vi "Get 3-Rayleigh Parameters(SubVI).vi"(6 "Flow Peak Amp.":dbl, 8 "T_Flow Start (s)":dbl, 9 "T_Flow Peak (s)":dbl, 10 "T_Ejection period (s)":dbl, 11 "Pressure (mmHg)":waveform(dbl)) -> (3 "Optimised Parameter":dbl[](array[numeric]))   [LabVIEW 2017]
uses:
  72fe1329-4430-4fd7-86c8-dfab2f7b2d2e.vi
  5c84d562-1cd3-438d-9587-7d7d9e0fcbf7.vi
panel:
  out "sorted 2D array":dbl[][](array[numeric])
  out "x-1":i32
  out "sorted array of params":dbl[][](array[numeric])
  out "Error Checks":dbl[][](array[numeric])
  out "Parameters":dbl[][](array[numeric])
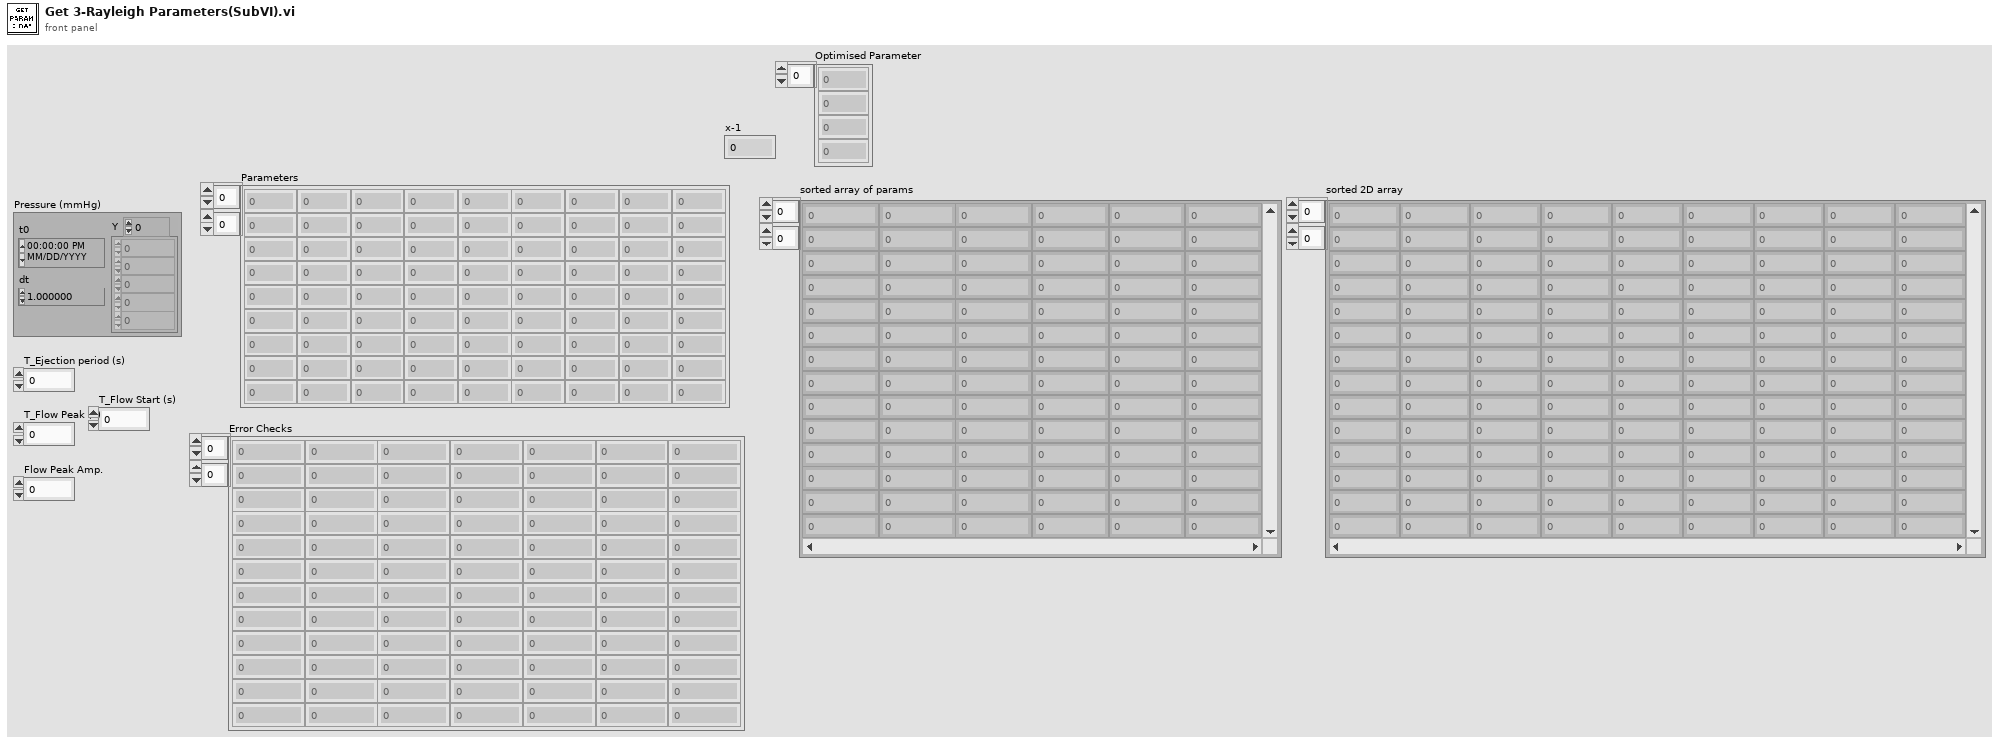
[diagram p1: front panel]
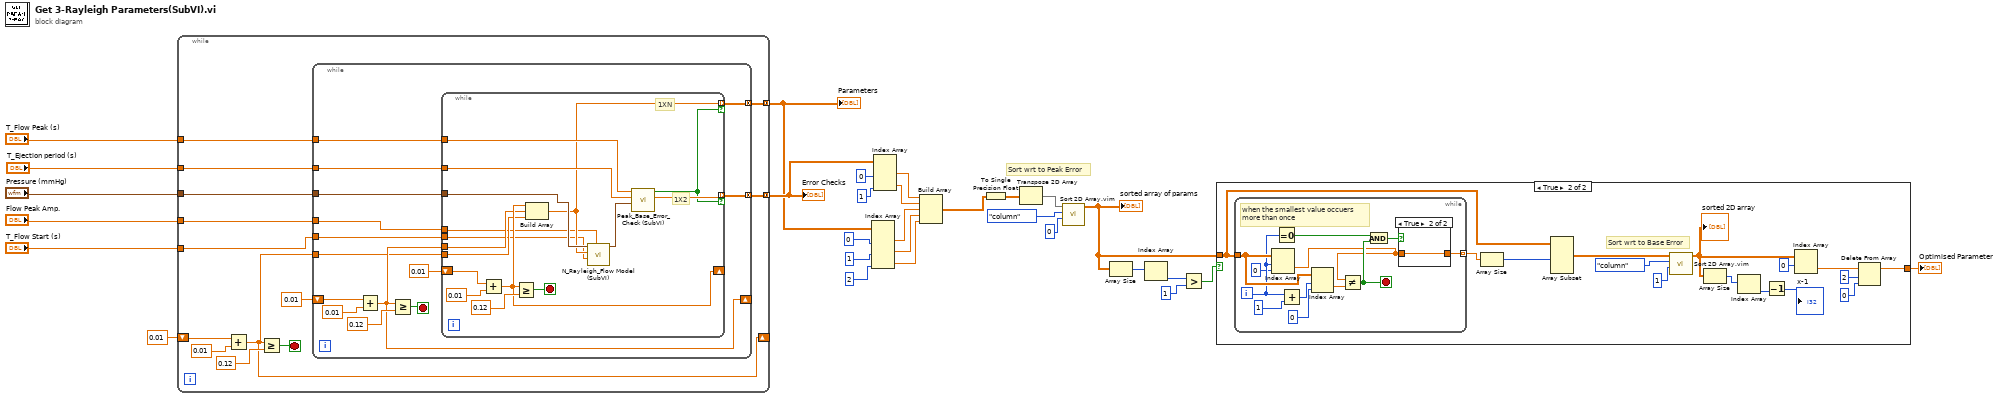
[diagram p0: block diagram]
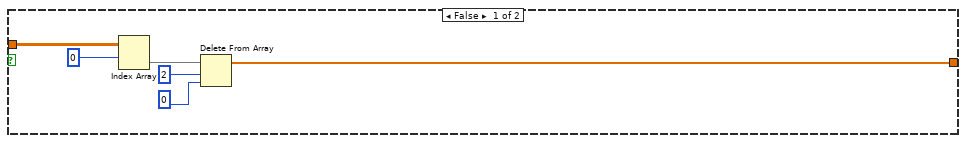
[diagram p2: hidden frame]
diagram:
  # "Sort wrt to Peak Error"
  n1 = while {
    tunnel: "Pressure (mmHg)" -> [w42]
    tunnel: "Flow Peak Amp." -> [w41]
    tunnel: "T_Ejection period (s)" -> [w39]
    tunnel: "T_Flow Peak (s)" -> [w38]
    tunnel: [w37] -> w19 mode=concatenating
    tunnel: [w36] -> w14 mode=concatenating
    tunnel: "T_Flow Start (s)" -> [w35]
    shift-right: [w30] -> _
    shift-left: 0.01 ("start") -> [w32]
    stop <- w31 stop-if-true
    n2 = Add(x=w32, y=0.01 ("start")) -> (x+y=w30:dbl)
    n3 = Greater Or Equal?(x=w30, y=0.12 ("start")) -> (x >= y?=w31:bool)
    n4 = while {
      tunnel: w42 -> [w56]
      tunnel: w41 -> [w55]
      shift-right: [w50] -> _
      shift-left: 0.01 ("start") -> [w53]
      tunnel: w39 -> [w48]
      tunnel: w38 -> [w47]
      tunnel: [w46] -> w36 mode=concatenating
      tunnel: [w45] -> w37 mode=concatenating
      tunnel: w35 -> [w44]
      tunnel: w30 -> [w43]
      stop <- w51 stop-if-true
      n5 = Add(x=w53, y=0.01 ("start")) -> (x+y=w50:dbl)
      n6 = Greater Or Equal?(x=w50, y=0.12 ("start")) -> (x >= y?=w51:bool)
      n7 = while {
        tunnel: w56 -> [w61]
        tunnel: w55 -> [w58]
        tunnel: w50 -> [w63]
        shift-right: [w64] -> _
        shift-left: 0.01 ("start") -> [w70]
        tunnel: w48 -> [w68]
        tunnel: w47 -> [w67]
        tunnel: [w60] -> w46 mode=indexing if=w65
        tunnel: [w66] -> w45 mode=indexing if=w65
        tunnel: w44 -> [w59]
        tunnel: w43 -> [w62]
        stop <- w69 stop-if-true
        # "1X2"
        # "1XN"
        n8 = Add(x=w70, y=0.01 ("start")) -> (x+y=w64:dbl)
        n9 = Greater Or Equal?(x=w64, y=0.12 ("start")) -> (x >= y?=w69:bool)
        n10 = Build Array(w64, w63, w62) -> (w60:dbl[])
        n11 = call "N_Rayleigh_Flow Model (SubVI).vi"("PSQ (ml/s)"=w58, "T_Flow Start"=w59, "Parameters (1XN)"=w60, "Pressure (mmHg)"=w61) -> ("n-Rayleigh Model Flow"=w57:waveform(dbl))  [unwired: 4 in, 1 out]
        n12 = call "Peak_Base_Error_Check (SubVI).vi"("Model Flow"=w57, "T_Ejection Period (s)"=w68, "T_Flow Peak (s)"=w67) -> ("Error"=w66:dbl[], "Logic"=w65:bool)  [unwired: 5 in, 2 out]
      }
    }
  }
  "Parameters" <- w14
  "Error Checks" <- w19
  n13 = Index Array(array=w14, index (col) #1=0 ("disabled index (col)"), index (col) #2=1 ("index (col)"), index (col) #3=2 ("index (col)")) -> (element #1=w16:dbl[], element #2=w15:dbl[], element #3=w1:dbl[])  [unwired: 3 in]
  n14 = Index Array(array=w19, index (col) #1=0 ("disabled index (col)"), index (col) #2=1 ("index (col)")) -> (element #1=w18:dbl[], element #2=w17:dbl[])  [unwired: 2 in]
  n15 = Build Array(w18, w17, w16, w15, w1) -> (w5:dbl[][])
  n16 = To Single Precision Float(number=w5) -> (single precision float=w6:sgl[][])
  n17 = Transpose 2D Array(2D array=w6) -> (transposed array=w13:sgl[][])
  n18 = call "Sort 2D Array.vim"("index"=0, "dimension to index (column)"=enum16{"column", "row"}."column", "2D array"=w13) -> ("sorted 2D array"=w7:sgl[][])  [unwired: 7 in, 1 out]
  "sorted array of params" <- w7
  n19 = Array Size(array=w7) -> (size(s)=w11:i32[])
  n20 = Index Array(array=w11) -> (element=w10:i32)  [unwired: 1 in]
  n21 = Greater?(x=w10, y=1) -> (0:w9:bool)
  n22 = case shown="True" w9 {
    tunnel: w7 -> [w78 w82]
    tunnel: [w73 w81] -> w8
    frame False {
      n23 = Index Array(array=w78, index (row)=0) -> (element=w76:sgl[])  [unwired: 1 in]
      n24 = Delete From Array(array=w76, length=2, index=0) -> (array with subset deleted=w73:sgl[])  [unwired: 1 out]
    }
    frame True {
      # "Sort wrt to Base Error"
      n25 = while {
        tunnel: w82 -> [w103]
        tunnel: [w100] -> w83 mode=indexing
        i -> [w102]
        stop <- w96 stop-if-true
        # "when the smallest value occuers \nmore than once"
        n26 = Index Array(array=w103, index (row)=w102, index (col)=0 ("disabled index (col)")) -> (element=w95:sgl)
        n27 = Equal To 0?(x=w102) -> (x = 0?=w101:bool)
        n28 = Add(x=w102, y=1) -> (x+y=w104:i32)
        n29 = Index Array(array=w103, index (row)=w104, index (col)=0 ("disabled index (col)")) -> (element=w94:sgl)
        n30 = Not Equal?(x=w95, y=w94) -> (x != y?=w96:bool)
        n31 = And(x=w101, y=w96) -> (x .and. y?=w97:bool)
        n32 = case shown="True" w97 {
          tunnel: w95 -> [w106 w107]
          tunnel: [w106 w107] -> w100
          frame False {
          }
          frame True {
          }
        }
      }
      n33 = Array Size(array=w83) -> (size(s)=w80:i32)
      n34 = Array Subset(array=w82, length (row)=w80) -> (w88:sgl[][])  [unwired: 3 in]
      n35 = call "Sort 2D Array.vim"("index"=1, "dimension to index (column)"=enum16{"column", "row"}."column", "2D array"=w88) -> ("sorted 2D array"=w89:sgl[][])  [unwired: 7 in, 1 out]
      "sorted 2D array" <- w89
      n36 = Array Size(array=w89) -> (size(s)=w90:i32[])
      n37 = Index Array(array=w90) -> (element=w91:i32)  [unwired: 1 in]
      n38 = Decrement(x=w91) -> (x-1=→"x-1":i32)
      n39 = Index Array(array=w89, index (row)=0) -> (element=w93:sgl[])  [unwired: 1 in]
      n40 = Delete From Array(array=w93, length=2, index=0) -> (array with subset deleted=w81:sgl[])  [unwired: 1 out]
    }
  }
  "Optimised Parameter" <- w8
